vi "Event_Generate.vi"(6 "Data":variant, 8 "error in (no error)":errorcluster, 9 "Parameter":string, 10 "Name":string, 11 "User Event in":T1) -> (0 "error out":errorcluster, 3 "User Event out":T1)   [LabVIEW 2020, in "hse-misc.lvlib"]
doc: "Generates an HSE-Event and sends <b>Name</b>, <b>Parameter</b> and <b>Data</b> as event data.\n\n\n\n____\nHAMPEL SOFTWARE ENGINEERING v3.8.0 (2023-12-18 14:41)"
uses:
  hse-misc.lvlib
  Event_GenericReference.ctl
  Event_GenericDatatype.ctl
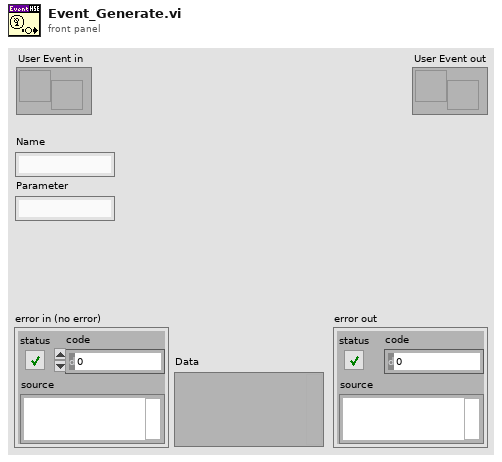
[diagram p1: front panel]
types:
  T1 = typedef "hse-misc.lvlib/Event_GenericReference.ctl" = refnum<user-event>
  T2 = typedef "hse-misc.lvlib/Event_GenericDatatype.ctl" = cluster{"name":string, "parameters":string, "data":variant}
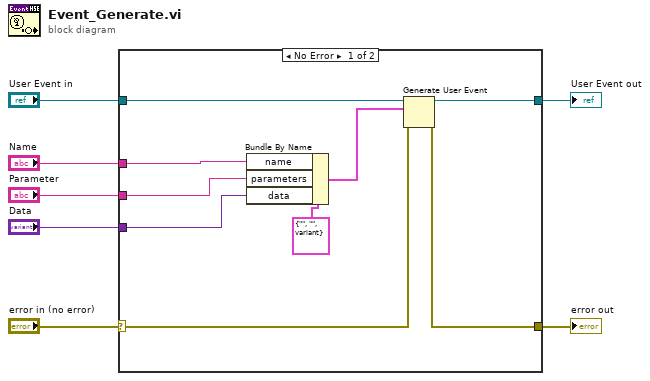
[diagram p0: block diagram]
diagram:
  n1 = case shown="No Error" "error in (no error)" {
    selector: "error in (no error)" -> [w9 w18]
    tunnel: "User Event in" -> [w16 w17]
    tunnel: [w15 w18] -> w6
    tunnel: "Name" -> [w13 _]
    tunnel: "Parameter" -> [w12 _]
    tunnel: "Data" -> [w11 _]
    tunnel: [w8 w17] -> w1
    frame No Error {
      n2 = Bundle By Name(cluster=T2 {"name"="", "parameters"="", "data"=variant} ("Event Datatype"), "name"=w13, "parameters"=w12, "data"=w11) -> (w10:T2)
      n3 = Generate User Event(user event=w16, event data cluster=w10, error in=w9) -> (user event out=w8:T1, error out=w15:errorcluster)  [unwired: 1 in]
    }
    frame Error {
    }
  }
  "error out" <- w6
  "User Event out" <- w1
